vi "test Fails If One String Is Empty and One Is Not.vi"(8 "error in (no error)":errorcluster, 11 "TestCase in":refnum<class "String Equality Test Case.lvclass">) -> (0 "error out":errorcluster, 3 "TestCase out":refnum<class "String Equality Test Case.lvclass">)   [LabVIEW 2015, in "String Equality Test Case.lvclass"]
uses:
  String Equality Test Case.lvclass
  <vilib>/addons/_JKI Toolkits/VI Tester/TestCase.llb/TestCase.lvclass
  VITAC.lvlib
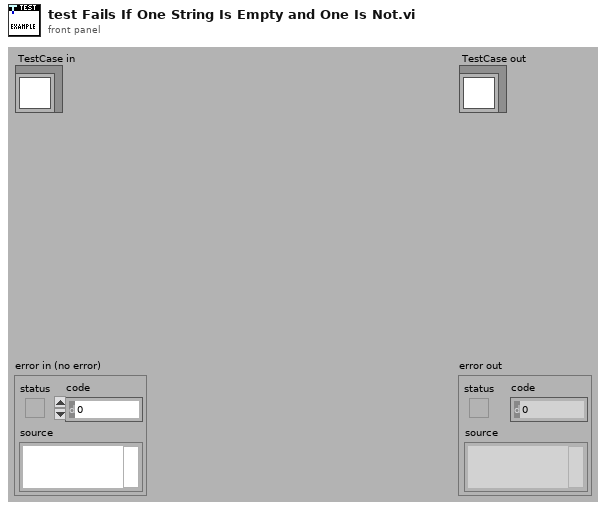
[diagram p1: front panel]
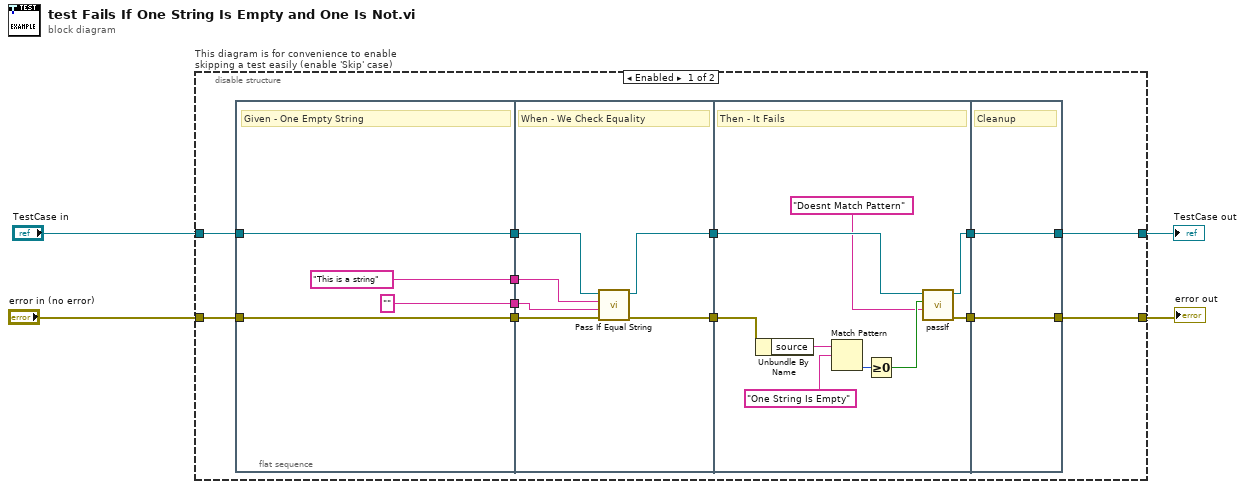
[diagram p0: block diagram]
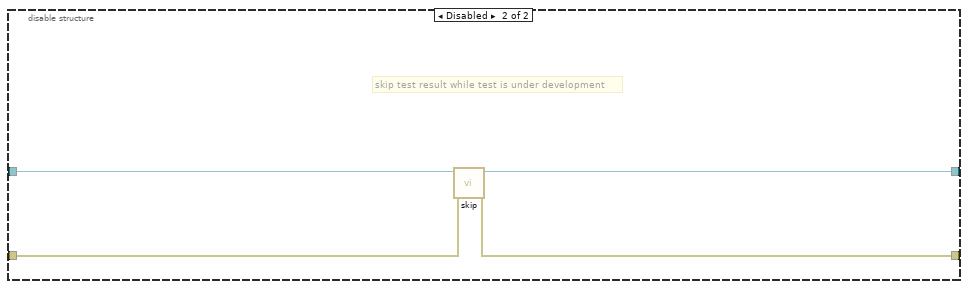
[diagram p2: hidden frame]
diagram:
  n1 = disable-structure "This diagram is for convenience to enable skipping a test easily (enable 'Skip' case)" shown="Enabled" {
    disable-tunnel: "TestCase in" -> [w16 w41]
    disable-tunnel: [w15 w39] -> w1
    disable-tunnel: [w14 w40] -> w3
    disable-tunnel: "error in (no error)" -> [w13 w38]
    frame Enabled {
      n2 = flat-sequence {
        tunnel: w13 -> [w19]
        tunnel: w16 -> [w20]
        tunnel: [w20] -> w8
        tunnel: [w19] -> w7
        tunnel: ["This is a string" ("expected")] -> w6
        tunnel: ["" ("expected")] -> w5
        tunnel: [w23] -> w10
        tunnel: [w25] -> w9
        tunnel: w8 -> [w24]
        tunnel: w7 -> [w26]
        tunnel: w6 -> [w22]
        tunnel: w5 -> [w21]
        tunnel: [w33] -> w12
        tunnel: [w35] -> w11
        tunnel: w10 -> [w34]
        tunnel: w9 -> [w32]
        tunnel: [w36] -> w14
        tunnel: [w37] -> w15
        tunnel: w12 -> [w37]
        tunnel: w11 -> [w36]
        frame #0 {
          # "Given - One Empty String"
        }
        frame #1 {
          # "When - We Check Equality"
          n3 = call "Pass If Equal String.vi"("error in (no error)"=w26, "actual"=w21, "expected"=w22, "TestCase in"=w24) -> ("error out"=w25:errorcluster, "TestCase out"=w23:refnum<class "String Equality Test Case.lvclass">)  [unwired: 6 in]
        }
        frame #2 {
          # "Then - It Fails"
          n4 = Unbundle By Name(w32) -> ("source"=w31:string)
          n5 = Match Pattern(string=w31, regular expression="One String Is Empty") -> (offset past match=w29:i32)  [unwired: 1 in, 3 out]
          n6 = Greater Or Equal To 0?(x=w29) -> (x >= 0?=w28:bool)
          n7 = call-dynamic "passIf.vi"("message (\"\")"="Doesnt Match Pattern" ("custom report message (\"\")"), "pass"=w28, "TestCase in"=w34) -> ("error out"=w35:errorcluster, "TestCase out"=w33:refnum<class "String Equality Test Case.lvclass">)  [unwired: 7 in]
        }
        frame #3 {
          # "Cleanup"
        }
      }
    }
    frame Disabled {
      # "skip test result while test is under development"
      n8 = call <vilib>:"skip.vi"("error in (no error)"=w38, "TestCase in"=w41) -> ("error out"=w40:errorcluster, "TestCase out"=w39:refnum<class "String Equality Test Case.lvclass">)  [unwired: 8 in]
    }
  }
  "error out" <- w3
  "TestCase out" <- w1
